vi "Translate_CartesianVector.vi"(7 "Translation Type":T1, 8 "error in (no error)":errorcluster, 10 "CartesianVector.lvclass":refnum<class "CartesianVector.lvclass">, 11 "PolarVector in":refnum<class "PolarVector.lvclass">) -> (0 "error out":errorcluster, 3 "PolarVector out":refnum<class "PolarVector.lvclass">)   [LabVIEW 2013, in "PolarVector.lvclass"]
doc: "Takes in a PolarVector object and a Cartesian Vector object as well as a translation type. Outputs a new PolarVector object that is the result of translating the input PolarVector object by the CartesianVector object."
uses:
  PolarVector.lvclass
  TypeDefs/TranslationType.ctl
  CartesianVector/CartesianVector.lvclass
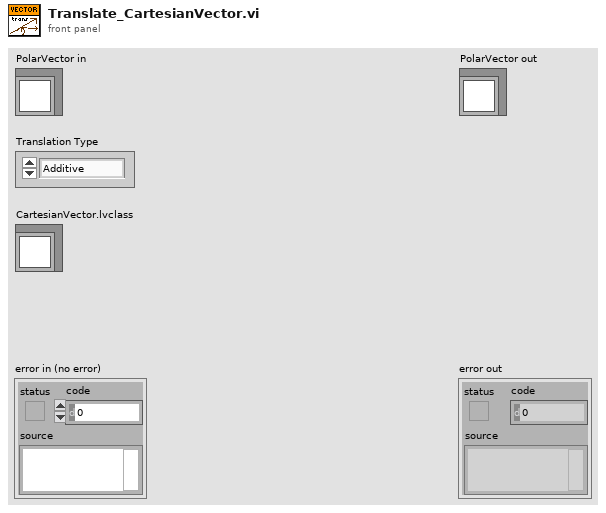
[diagram p1: front panel]
types:
  T1 = typedef "TranslationType.ctl" = enum16{"Additive", "Subtractive"}
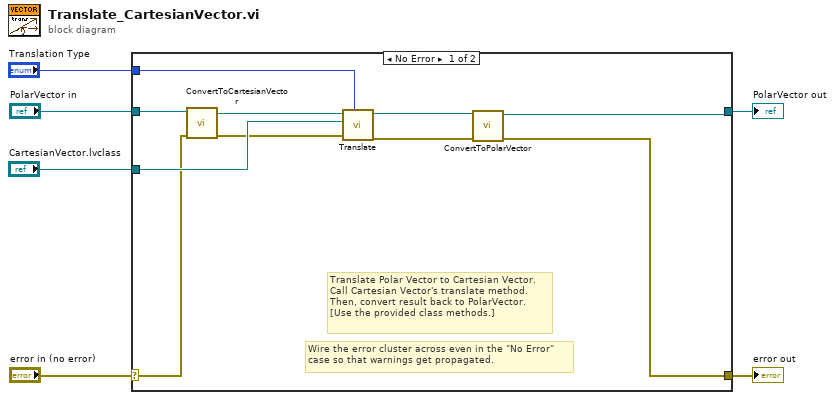
[diagram p0: block diagram]
diagram:
  n1 = case shown="No Error" "error in (no error)" {
    selector: "error in (no error)" -> [w13 w18]
    tunnel: [w7 w18] -> w5
    tunnel: [w8 w17] -> w3
    tunnel: "PolarVector in" -> [w16 w17]
    tunnel: "CartesianVector.lvclass" -> [w14 _]
    tunnel: "Translation Type" -> [w11 _]
    frame No Error {
      # "Translate Polar Vector to Cartesian Vector.\nCall Cartesian Vector's translate method.\nThen, convert result back to PolarVector.\n[Use the provided class methods.]"
      # "Wire the error cluster across even in the \"No Error\"\ncase so that warnings get propagated."
      n2 = call "ConvertToCartesianVector.vi"("error in (no error)"=w13, "PolarVector in"=w16) -> ("error out"=w12:errorcluster, "CartesianVector.lvclass"=w15:refnum<class "CartesianVector.lvclass">)  [unwired: 8 in]
      n3 = call-poly "Translate.vi"("Translation Type"=w11, "error in (no error)"=w12, "CV 2"=w14, "CV 1"=w15) -> ("error out"=w9:errorcluster, "CV 1 Translated by CV 2"=w10:refnum<class "CartesianVector.lvclass">)  [unwired: 6 in]
      n4 = call "ConvertToPolarVector.vi"("error in (no error)"=w9, "CartesianVector in"=w10) -> ("error out"=w7:errorcluster, "PolarVector.lvclass"=w8:refnum<class "PolarVector.lvclass">)  [unwired: 8 in]
    }
    frame Error {
    }
  }
  "error out" <- w5
  "PolarVector out" <- w3
